vi "Calculate ramp power.vi"(8 "error in (no error)":errorcluster, 9 "Time between updates (ms)":i32, 10 "Current update":i32, 11 "AOTF in":refnum<class "AOTF.lvclass">) -> (0 "error out":errorcluster, 2 "finished?":bool, 3 "AOTF out":refnum<class "AOTF.lvclass">)   [LabVIEW 2012, in "AOTF.lvclass"]
uses:
  AOTF.lvclass
  AOTF.lvclass/AOTF.ctl
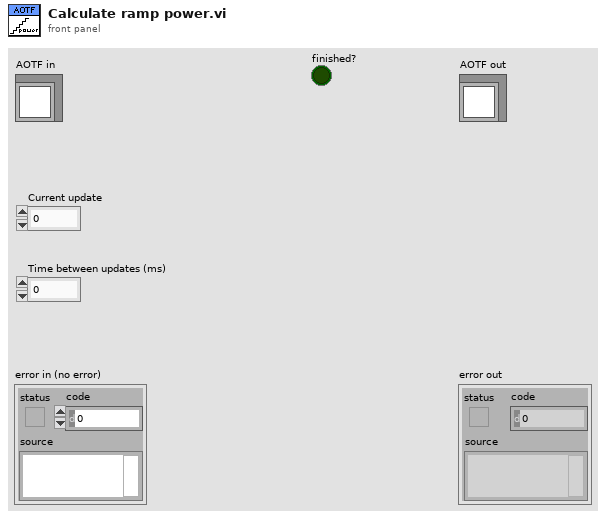
[diagram p1: front panel]
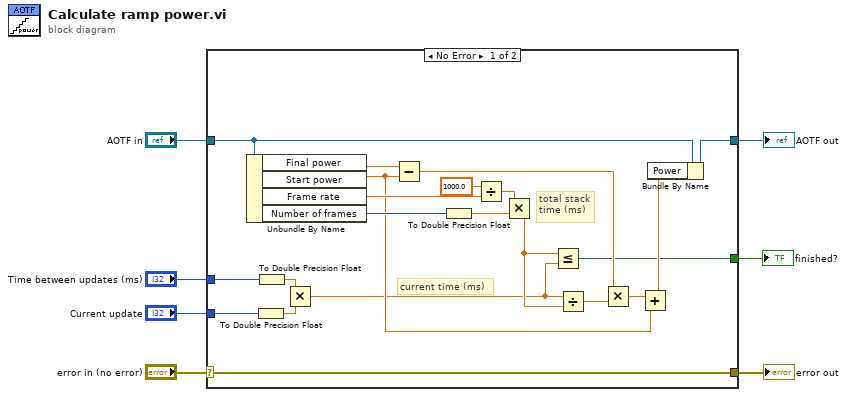
[diagram p0: block diagram]
diagram:
  n1 = case shown="No Error" "error in (no error)" {
    selector: "error in (no error)" -> [w28 w30]
    tunnel: [w28 w30] -> w6
    tunnel: [w26 w29] -> w4
    tunnel: "AOTF in" -> [w27 w29]
    tunnel: "Time between updates (ms)" -> [w19 _]
    tunnel: "Current update" -> [w18 _]
    tunnel: [w8 _] -> w1
    frame No Error {
      # "current time (ms)"
      # "total stack\ntime (ms)"
      n2 = Unbundle By Name(w27) -> ("Final power"=w25:dbl, "Start power"=w12:dbl, "Frame rate"=w24:dbl, "Number of frames"=w21:i32)
      n3 = To Double Precision Float(number=w18) -> (double precision float=w17:dbl)
      n4 = To Double Precision Float(number=w19) -> (double precision float=w16:dbl)
      n5 = Multiply(x=w16, y=w17) -> (x*y=w9:dbl)
      n6 = Subtract(x=w25, y=w12) -> (x-y=w14:dbl)
      n7 = To Double Precision Float(number=w21) -> (double precision float=w20:dbl)
      n8 = Divide(x=1000.0, y=w24) -> (x/y=w22:dbl)
      n9 = Multiply(x=w22, y=w20) -> (x*y=w10:dbl)
      n10 = Less Or Equal?(x=w10, y=w9) -> (x <= y?=w8:bool)
      n11 = Divide(x=w9, y=w10) -> (x/y=w15:dbl)
      n12 = Multiply(x=w14, y=w15) -> (x*y=w13:dbl)
      n13 = Add(x=w13, y=w12) -> (x+y=w11:dbl)
      n14 = Bundle By Name(cluster=w27, "Power"=w11) -> (w26:refnum<class "AOTF.lvclass">)
    }
    frame Error {
    }
  }
  "error out" <- w6
  "AOTF out" <- w4
  "finished?" <- w1
